vi "Launch New Task.vi"(8 "error in (no error)":errorcluster, 9 "Timeout mS (10000)":i32=10000, 10 "Task":refnum<class "Task.lvclass">, 11 "VolatusAPI in":refnum<class "VolatusAPI.lvclass">) -> (0 "error out":errorcluster, 2 "EnQr":refnum<class "Message Enqueuer.lvclass">, 3 "VolatusAPI out":refnum<class "VolatusAPI.lvclass">)   [LabVIEW 2020, in "Volatus.lvlib" / "VolatusAPI.lvclass"]
uses:
  VolatusAPI.lvclass
  Task/Task.lvclass
  <vilib>/ActorFramework/Message Enqueuer/Message Enqueuer.lvclass
  TaskEnQrValue/TaskEnQrValue.lvclass
  C:/dev/lv20CE/relink/lv-promises/Promises/Value/Value.lvclass
  VolatusAPI.lvclass/VolatusAPI.ctl
  lv-promises/Promises/Promise/Promise.lvclass/Promise.ctl
  lv-promises/Promises/Future/Future.lvclass/Future.ctl
  VolatusCoreTask Messages/Launch New Task Msg/Launch New Task Msg.lvclass/Launch New Task Msg.ctl
  <vilib>/ActorFramework/Message Enqueuer/Message Enqueuer.lvclass/Message Enqueuer.ctl
  <vilib>/ActorFramework/Message Enqueuer/Enqueue.vi
  VolatusCoreTask Messages/Launch New Task Msg/Launch New Task Msg.lvclass
  C:/Program Files (x86)/National Instruments/LabVIEW 2020/vi.lib/ActorFramework/Message/Message.lvclass
  <vilib>/ActorFramework/Message Priority Queue/Priority Enqueue.vi
  lv-promises/Promises/Future/Future.lvclass
  lv-promises/Promises/Promise/Promise.lvclass
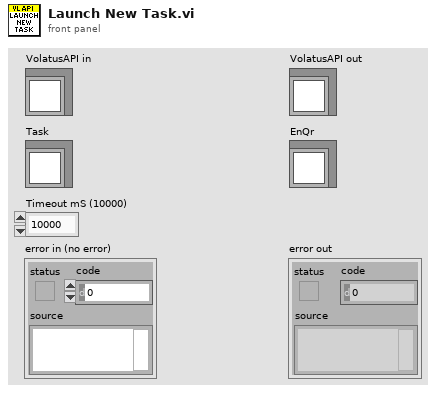
[diagram p1: front panel]
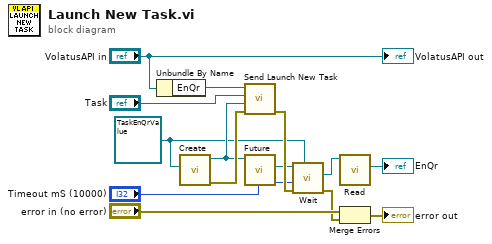
[diagram p0: block diagram]
diagram:
  w5 = refnum<class "TaskEnQrValue.lvclass"> refnum ("Volatus:TaskEnQrValue.lvclass")
  n1 = Unbundle By Name("VolatusAPI in") -> ("EnQr"=w11:refnum<class "Message Enqueuer.lvclass">)
  n2 = call "Create.vi"("Result Type"=w5) -> ("error out"=w9:errorcluster, "Promise"=w8:refnum<class "Promise.lvclass">)  [unwired: 9 in]
  n3 = call "Send Launch New Task.vi"("error in (no error)"=w9, "Promise"=w8, "Task"="Task", "Message Enqueuer"=w11) -> ("error out"=w14:errorcluster)  [unwired: 6 in, 1 out]
  n4 = call "Future.vi"("Promise in"=w8) -> ("Future"=w7:refnum<class "Future.lvclass">)  [unwired: 9 in, 1 out]
  n5 = call "Wait.vi"("Result Type"=w5, "error in (no error)"=w14, "Timeout mS (-1)"="Timeout mS (10000)", "Future in"=w7) -> ("error out"=w1:errorcluster, "Result"=w4:refnum<class "TaskEnQrValue.lvclass">)  [unwired: 6 in]
  n6 = call "Read.vi"("TaskEnQrValue in"=w4) -> ("EnQr"=→"EnQr":refnum<class "Message Enqueuer.lvclass">)  [unwired: 10 in]
  n7 = Merge Errors("error in (no error)", w1) -> (→"error out":errorcluster)
  "VolatusAPI out" <- "VolatusAPI in"
